vi "水果摊贩子_main.vi"() -> ()   [LabVIEW 2011]
uses:
  <vilib>/Utility/file.llb/Read From Spreadsheet File (string).vi
panel:
  in  "富豪榜":i32[](listbox)
  out "leave":bool
  in  "关闭富豪榜":bool
  in  "查看富豪榜":bool
  in  "退出？":bool
  out "玩家":string caption="请输入你的大名"
  in  "放弃游戏":bool
  out "开心值":dbl(slide) scale=0.0..100.0
  out "当前开心值":i32=1000
  out "提示":string
  in  "银行":bool
  out "存款":i32
  in  "演会中心":bool
  in  "机电学院":bool
  out "天数":i32
  out "余额":i32
  in  "饭堂":bool
  in  "图书馆":bool
  in  "库存":i32[](listbox)
  in  "卖出数量":i32 min=0 step=1
  in  "买入数量":i32 min=0 step=1
  in  "卖出":bool
  in  "买入":bool
  in  "商品价格":i32[](listbox)
  out "物品存在索引":i32[](array[numeric])
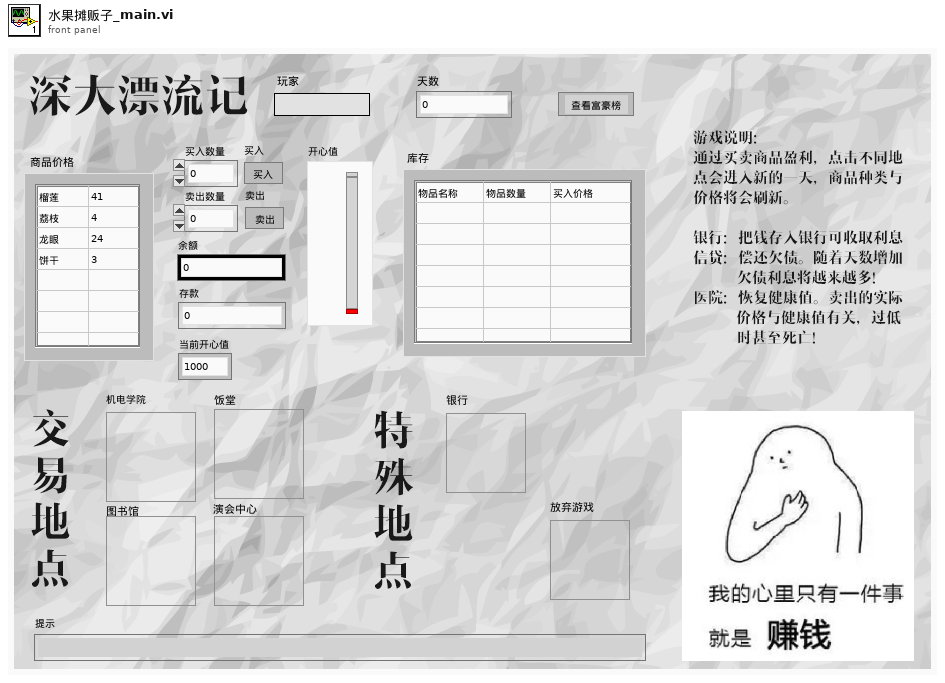
[diagram p1: front panel]
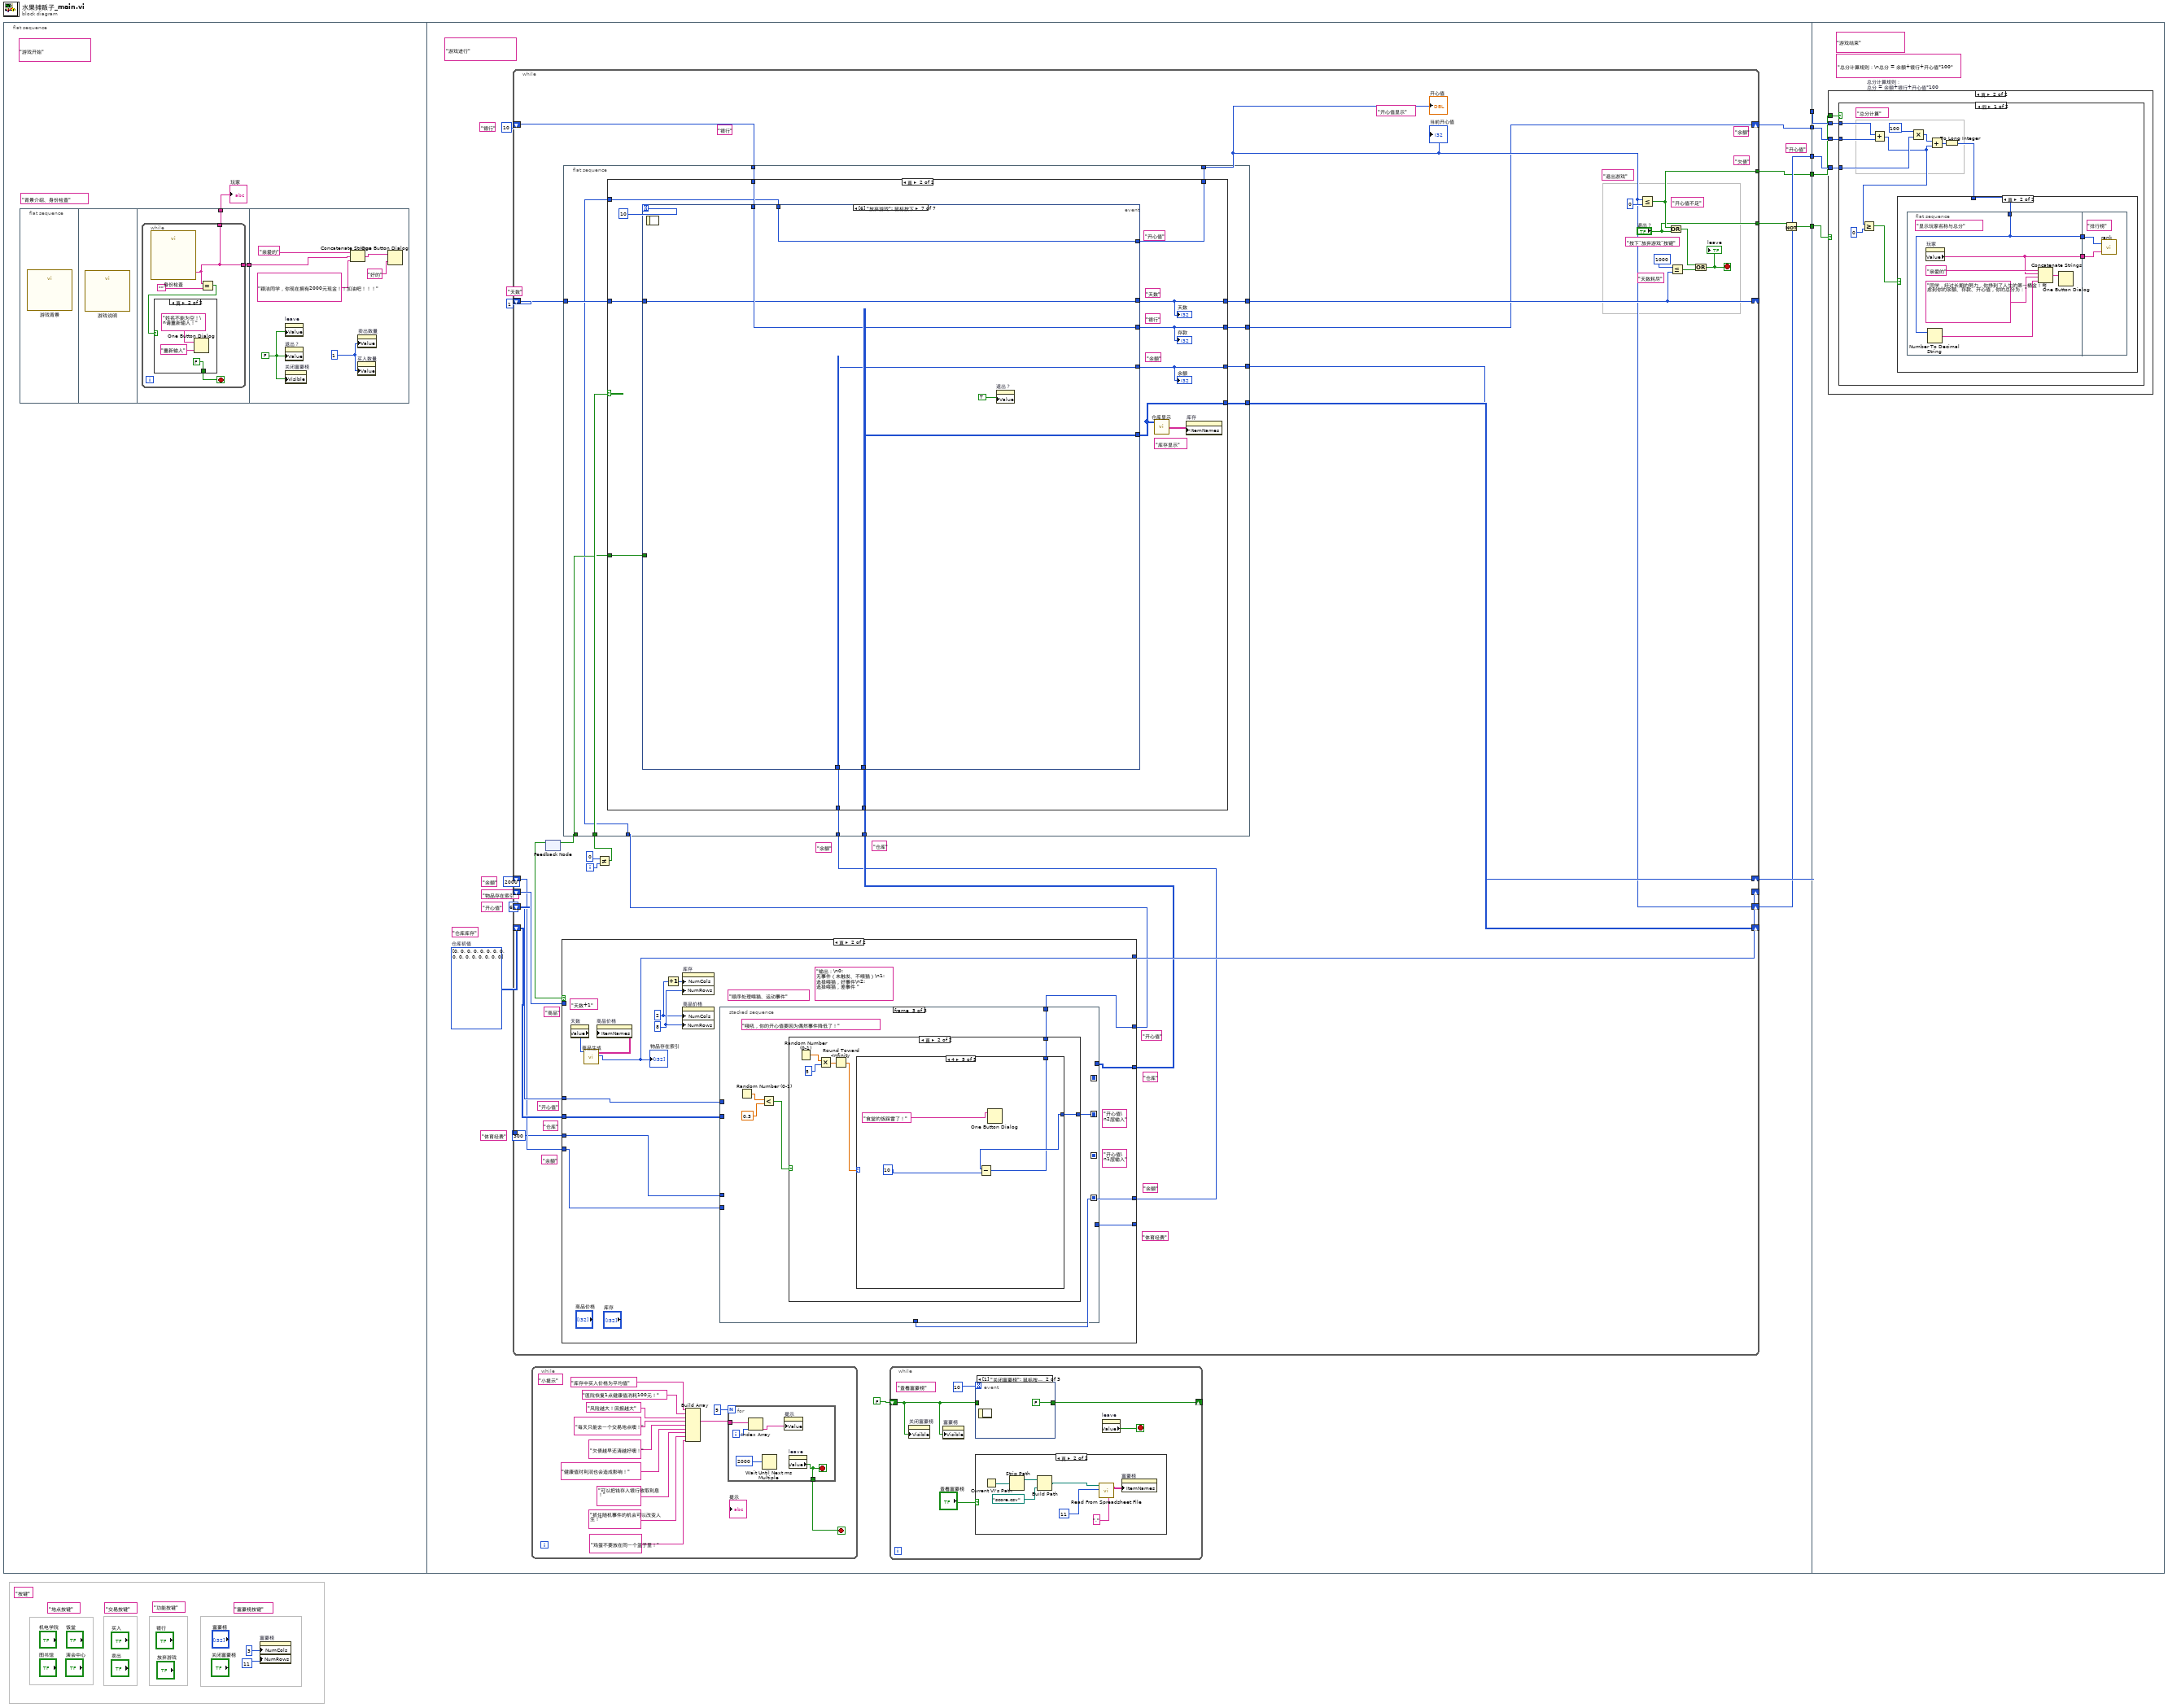
[diagram p0: block diagram]
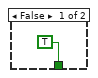
[diagram p2: hidden frame]
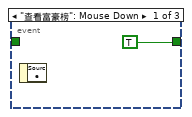
[diagram p3: hidden frame]
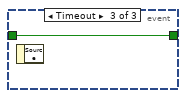
[diagram p4: hidden frame]
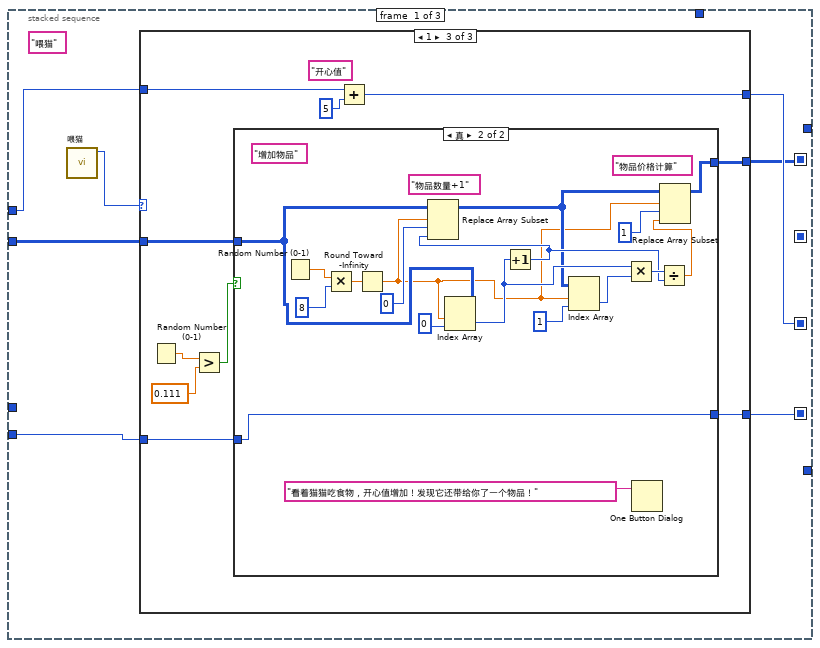
[diagram p7: hidden frame]
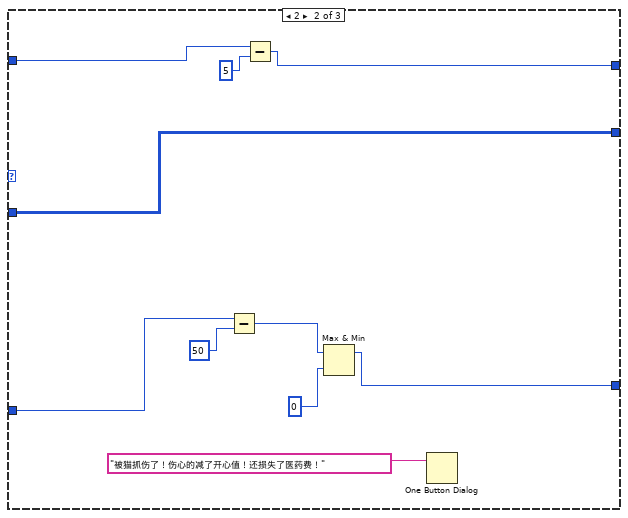
[diagram p9: hidden frame]
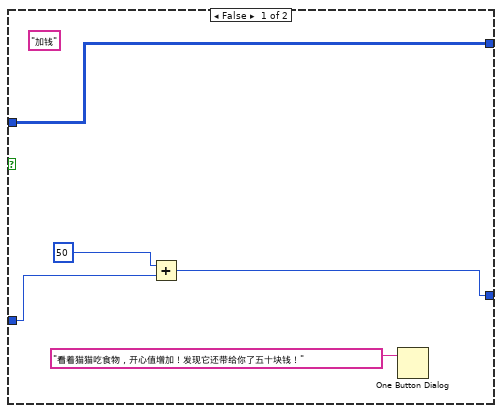
[diagram p10: hidden frame]
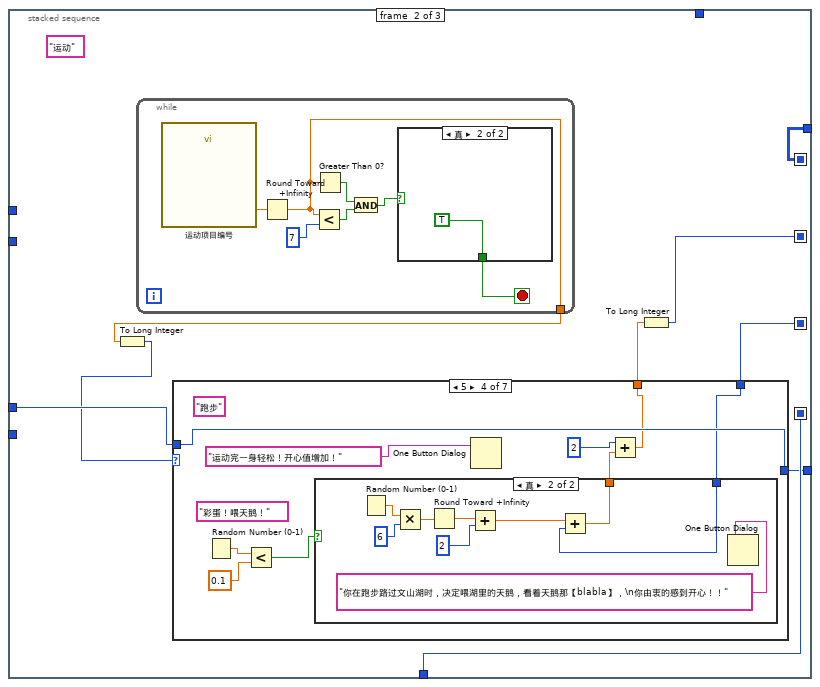
[diagram p11: hidden frame]
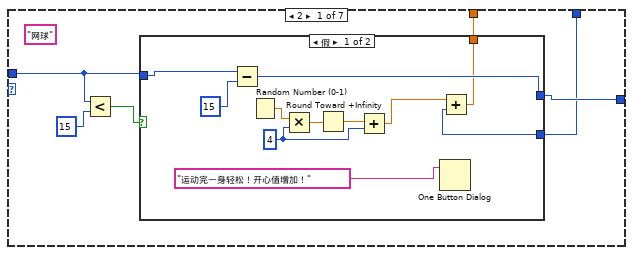
[diagram p12: hidden frame]
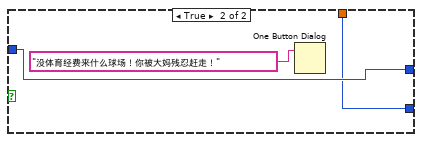
[diagram p13: hidden frame]
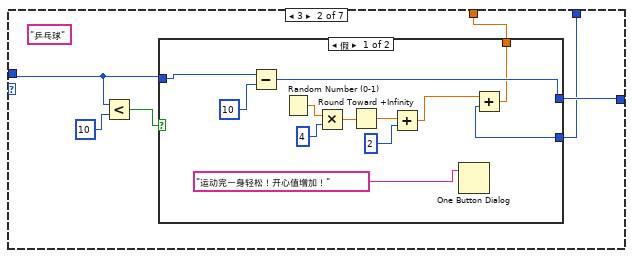
[diagram p14: hidden frame]
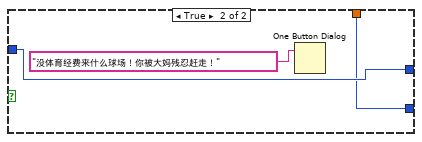
[diagram p15: hidden frame]
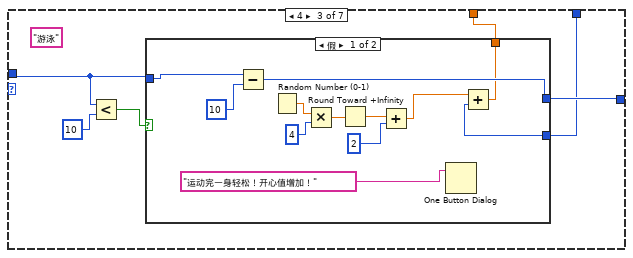
[diagram p16: hidden frame]
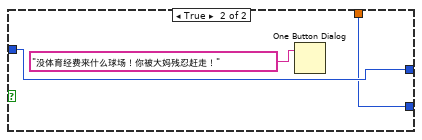
[diagram p17: hidden frame]
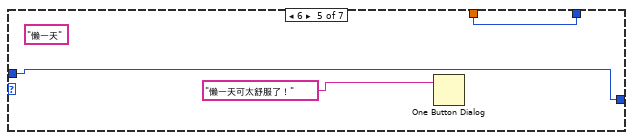
[diagram p19: hidden frame]
diagram:
  (unwired) "富豪榜按键"
  (unwired) "功能按键"
  (unwired) "交易按键"
  (unwired) "地点按键"
  (unwired) "按键"
  n1 = flat-sequence {
    tunnel: [w39] -> w7
    tunnel: [w38] -> w6
    tunnel: [w37] -> w5
    tunnel: [w36] -> w4
    tunnel: [w28] -> w1
    tunnel: w7 -> [w656]
    tunnel: w6 -> [w655]
    tunnel: w5 -> [w654]
    tunnel: w4 -> [w653]
    tunnel: w1 -> [w652]
    frame #0 {
      (unwired) "背景介绍、身份检查"
      (unwired) "游戏开始"
      n2 = flat-sequence {
        tunnel: [w11] -> w9
        tunnel: [w10] -> w8
        tunnel: w9 -> [w25]
        frame #0 {
          n3 = call "游戏背景"() -> ()  [unwired: 18 in, 2 out]
        }
        frame #1 {
          n4 = call "游戏说明"() -> ()  [unwired: 18 in, 2 out]
        }
        frame #2 {
          n5 = while {
            tunnel: [w12] -> w11
            tunnel: [w12] -> w10
            stop <- w13 stop-if-true
            n6 = call "身份检查"() -> ("请输入你的姓名"=w12:string)  [unwired: 17 in, 2 out]
            n7 = Equal?(x=w12, y="") -> (x = y?=w14:bool)
            n8 = case shown="真" w14 {
              tunnel: [TRUE FALSE] -> w13
              frame False {
              }
              frame True {
                n9 = One Button Dialog(message="姓名不能为空！\n请重新输入！", button name ("OK")="重新输入" ("姓名输入提示")) -> ()  [unwired: 1 out]
              }
            }
          }
        }
        frame #3 {
          w20 = 1
          w21 = FALSE
          n10 = property on="leave" class="Bool (严格)"("Value"=w21) -> ()  [unwired: 2 in, 2 out]
          n11 = property on="退出？" class="Bool (严格)"("Value"=w21) -> ()  [unwired: 2 in, 2 out]
          n12 = property on="关闭富豪榜" class="Bool (严格)"("Visible"=w21) -> ()  [unwired: 2 in, 2 out]
          n13 = Concatenate Strings("亲爱的" ("姓名输入提示"), w25, "颖洁同学，你现在拥有2000元现金！！加油吧！！！" ("姓名输入提示")) -> (w23:string)
          n14 = property on="买入数量" class="DigNum (严格)"("Value"=w20) -> ()  [unwired: 2 in, 2 out]
          n15 = property on="卖出数量" class="DigNum (严格)"("Value"=w20) -> ()  [unwired: 2 in, 2 out]
          n16 = One Button Dialog(message=w23, button name ("OK")="好的" ("姓名输入提示")) -> ()  [unwired: 1 out]
        }
      }
      "玩家" <- w8
    }
    frame #1 {
      (unwired) "开心值"
      (unwired) "体育经费"
      (unwired) "物品存在索引"
      (unwired) "游戏进行"
      (unwired) "开心值"
      (unwired) "银行"
      (unwired) "仓库库存"
      (unwired) "天数"
      (unwired) "余额"
      w32 = i32[][] [[0, 0], [0, 0], [0, 0], [0, 0], [0, 0], [0, 0], [0, 0], [0, 0]]  # 仓库初值
      n17 = while {
        shift-right: [w94] -> w39
        shift-left: 2000 -> [w75]
        shift-right: [w95] -> _
        shift-left: w32 -> [w77]
        shift-right: [w98] -> _
        shift-left: _ -> [w97]
        shift-right: [w91] -> _
        shift-left: 1 -> [w88]
        shift-right: [w81] -> w38
        shift-left: 10 -> [w89]
        shift-right: [w82] -> w37
        shift-left: 60 -> [w90]
        tunnel: [w83] -> w36
        tunnel: ["退出？"] -> w29
        tunnel: 300 -> [w72]
        i -> [w93]
        stop <- w86 stop-if-true
        (unwired) "仓库"
        (unwired) "体育经费"
        (unwired) "仓库"
        (unwired) "开心值"
        (unwired) "余额"
        (unwired) "余额"
        (unwired) "天数耗尽"
        (unwired) "按下“放弃游戏”按键"
        (unwired) "开心值不足"
        (unwired) "退出游戏"
        (unwired) "开心值显示"
        (unwired) "开心值"
        (unwired) "余额"
        (unwired) "欠债"
        (unwired) "商品"
        (unwired) "仓库"
        (unwired) "余额"
        (unwired) "银行"
        n18 = feedback-in #1(w80) -> ()
        n19 = feedback #1() -> (w96:bool)  [unwired: 1 in]
        n20 = case shown="真" w96 {
          tunnel: [w104 w114] -> w98
          tunnel: w97 -> [w104 _]
          tunnel: w90 -> [w103 w105]
          tunnel: [w103 w112] -> w73
          tunnel: w77 -> [w102 w111]
          tunnel: [w102 w108] -> w76
          tunnel: w75 -> [w101 w110]
          tunnel: [w101 w109] -> w74
          tunnel: w72 -> [w100 w107]
          tunnel: [w100 w106] -> _
          frame False {
          }
          frame True {
            (unwired) "开心值\n2层输入"
            (unwired) "开心值\n1层输入"
            (unwired) "输出：\n0: 无事件（未触发、不喂猫）\n1: 选择喂猫，好事件\n2: 选择喂猫，差事件 "
            (unwired) "顺序处理喂猫、运动事件"
            (unwired) "天数+1"
            w118 = i8 8
            w116 = i8 2
            n21 = property on="天数" class="DigNum (严格)"() -> ("Value"=w113:i32)  [unwired: 2 in, 2 out]
            n22 = call "商品生成.vi"("天数"=w113) -> ("物品存在索引"=w114:i32[], "市面商品"=w115:string[][])  [unwired: 9 in]
            "物品存在索引" <- w114
            n23 = property on="商品价格" class="MCListbox (严格)"("ItemNames"=w115) -> ()  [unwired: 2 in, 2 out]
            n24 = Increment(x=w116) -> (x+1=w117:i8)
            n25 = property on="库存" class="MCListbox (严格)"("NumCols"=w117, "NumRows"=w118) -> ()  [unwired: 2 in, 2 out]
            n26 = property on="商品价格" class="MCListbox (严格)"("NumCols"=w116, "NumRows"=w118) -> ()  [unwired: 2 in, 2 out]
            n27 = stacked-sequence {
              seq-local: [w124 _ _] -> [_ w177 _]
              seq-local: [w122 _ _] -> [_ w174 _]
              seq-local: [w119 _ _] -> [_ w180 _]
              seq-local: [_ w175 _] -> [_ _ w299]
              tunnel: w105 -> [w125 _ _]
              tunnel: w111 -> [w123 _ _]
              tunnel: w110 -> [w120 _ _]
              tunnel: [_ _ w298] -> w112
              tunnel: [_ w180 _] -> w109
              tunnel: [_ w174 _] -> w108
              tunnel: w107 -> [_ w179 _]
              tunnel: [_ w178 _] -> w106
              frame #0 {
                (unwired) "喂猫"
                n28 = call "喂猫.vi"() -> ("数值"=w121:i8)  [unwired: 11 in]
                n29 = case shown="1" w121 {
                  tunnel: w125 -> [w128 w137 w147]
                  tunnel: [w128 w136 w146] -> w124
                  tunnel: w123 -> [w127 w135 w145]
                  tunnel: [w127 w135 w144] -> w122
                  tunnel: w120 -> [w126 w133 w140]
                  tunnel: [w126 w130 w139] -> w119
                  frame 0, Default {
                  }
                  frame 2 {
                    n30 = Subtract(x=w133, y=50) -> (x-y=w131:i32)
                    n31 = Subtract(x=w137, y=5) -> (x-y=w136:i32)
                    n32 = Max & Min(x=w131, y=0) -> (max(x,y)=w130:i32)  [unwired: 1 out]
                    n33 = One Button Dialog(message="被猫抓伤了！伤心的减了开心值！还损失了医药费！") -> ()  [unwired: 1 in, 1 out]
                  }
                  frame 1 {
                    (unwired) "开心值"
                    n34 = Random Number (0-1)() -> (number: 0 to 1=w143:dbl)
                    n35 = Greater?(x=w143, y=0.111) -> (0:w141:bool)
                    n36 = case shown="真" w141 {
                      tunnel: w145 -> [w153 w166]
                      tunnel: [w153 w156] -> w144
                      tunnel: w140 -> [w152 w155]
                      tunnel: [w150 w155] -> w139
                      frame False {
                        (unwired) "加钱"
                        n37 = Add(x=50, y=w152) -> (x+y=w150:i32)
                        n38 = One Button Dialog(message="看着猫猫吃食物，开心值增加！发现它还带给你了五十块钱！") -> ()  [unwired: 1 in, 1 out]
                      }
                      frame True {
                        (unwired) "物品价格计算"
                        (unwired) "物品数量+1"
                        (unwired) "增加物品"
                        n39 = Random Number (0-1)() -> (number: 0 to 1=w171:dbl)
                        n40 = Multiply(x=w171, y=8) -> (x*y=w169:dbl)
                        n41 = Round Toward -Infinity(1:w169) -> (0:w159:dbl)
                        n42 = Index Array(array=w166, index (row)=w159, index (col)=0) -> (element=w164:i32)
                        n43 = Increment(x=w164) -> (x+1=w161:i32)
                        n44 = Replace Array Subset ("替换数组子集")(array=w166, new element=w161, index (row)=w159, index (col)=0) -> (w160:i32[][])
                        n45 = Index Array(array=w160, index (row)=w159, index (col)=1) -> (element=w167:i32)
                        n46 = Multiply(x=w164, y=w167) -> (x*y=w162:i32)
                        n47 = One Button Dialog(message="看着猫猫吃食物，开心值增加！发现它还带给你了一个物品！") -> ()  [unwired: 1 in, 1 out]
                        n48 = Divide(x=w162, y=w161) -> (x/y=w157:dbl)
                        n49 = Replace Array Subset ("替换数组子集")(array=w160, new element=w157, index (row)=w159, index (col)=1) -> (w156:i32[][])
                      }
                    }
                    n50 = Add(x=w147, y=5) -> (x+y=w146:i32)
                  }
                }
              }
              frame #1 {
                (unwired) "运动"
                n51 = while {
                  tunnel: [w287] -> w173
                  stop <- w288 stop-if-true
                  n52 = call "运动项目编号"() -> ("运动项目"=w293:dbl)  [unwired: 17 in, 2 out]
                  n53 = Round Toward +Infinity(x=w293) -> (ceil(x): smallest int >= x=w287:dbl)
                  n54 = Less?(x=w287, y=7) -> (x < y?=w291:bool)
                  n55 = Greater Than 0?(x=w287) -> (x > 0?=w290:bool)
                  n56 = And(x=w290, y=w291) -> (x .and. y?=w289:bool)
                  n57 = case shown="真" w289 {
                    tunnel: [FALSE TRUE] -> w288
                    frame False {
                      n58 = One Button Dialog(message="输入必须是1-7的整数！", button name ("OK")="重新输入" ("姓名输入提示")) -> ()  [unwired: 1 out]
                    }
                    frame True {
                    }
                  }
                }
                n59 = To Long Integer(number=w173) -> (32bit integer=w172:i32)
                n60 = case shown="5" w172 {
                  tunnel: w179 -> [w183 w203 w224 w251 w263 w265 w269]
                  tunnel: [w184 w204 w225 w251 w263 w265 w270] -> w178
                  tunnel: w177 -> [w182 w202 w223 w246 w262 w266 w268]
                  tunnel: [w181 w201 w222 w243 w262 w266 w267] -> w176
                  frame 2 {
                    (unwired) "网球" ("姓名输入提示")
                    n61 = Less?(x=w183, y=15) -> (x < y?=w185:bool)
                    n62 = case shown="假" w185 {
                      tunnel: w183 -> [w195 w199]
                      tunnel: [w194 w199] -> w184
                      tunnel: w182 -> [w188 w198]
                      tunnel: [w187 w198] -> w181
                      frame False {
                        w190 = 4
                        n63 = Subtract(x=w195, y=15) -> (x-y=w194:i32)
                        n64 = Random Number (0-1)() -> (number: 0 to 1=w193:dbl)
                        n65 = Multiply(x=w193, y=w190) -> (x*y=w192:dbl)
                        n66 = Round Toward +Infinity(x=w192) -> (ceil(x): smallest int >= x=w191:dbl)
                        n67 = Add(x=w191, y=w190) -> (x+y=w189:dbl)
                        n68 = One Button Dialog(message="运动完一身轻松！开心值增加！") -> ()  [unwired: 1 in, 1 out]
                        n69 = Add(x=w189, y=w188) -> (x+y=w187:dbl)
                      }
                      frame True {
                        n70 = One Button Dialog(message="没体育经费来什么球场！你被大妈残忍赶走！") -> ()  [unwired: 1 in, 1 out]
                      }
                    }
                  }
                  frame 3 {
                    (unwired) "乒乓球" ("姓名输入提示")
                    n71 = Less?(x=w203, y=10) -> (x < y?=w206:bool)
                    n72 = case shown="假" w206 {
                      tunnel: w203 -> [w216 w220]
                      tunnel: [w215 w220] -> w204
                      tunnel: w202 -> [w209 w219]
                      tunnel: [w208 w219] -> w201
                      frame False {
                        n73 = Subtract(x=w216, y=10) -> (x-y=w215:i32)
                        n74 = Random Number (0-1)() -> (number: 0 to 1=w214:dbl)
                        n75 = Multiply(x=w214, y=4) -> (x*y=w213:dbl)
                        n76 = Round Toward +Infinity(x=w213) -> (ceil(x): smallest int >= x=w212:dbl)
                        n77 = Add(x=w212, y=2) -> (x+y=w210:dbl)
                        n78 = One Button Dialog(message="运动完一身轻松！开心值增加！") -> ()  [unwired: 1 in, 1 out]
                        n79 = Add(x=w210, y=w209) -> (x+y=w208:dbl)
                      }
                      frame True {
                        n80 = One Button Dialog(message="没体育经费来什么球场！你被大妈残忍赶走！") -> ()  [unwired: 1 in, 1 out]
                      }
                    }
                  }
                  frame 4 {
                    (unwired) "游泳" ("姓名输入提示")
                    n81 = Less?(x=w224, y=10) -> (x < y?=w226:bool)
                    n82 = case shown="假" w226 {
                      tunnel: w224 -> [w237 w241]
                      tunnel: [w236 w241] -> w225
                      tunnel: w223 -> [w230 w240]
                      tunnel: [w229 w240] -> w222
                      frame False {
                        n83 = Subtract(x=w237, y=10) -> (x-y=w236:i32)
                        n84 = Random Number (0-1)() -> (number: 0 to 1=w235:dbl)
                        n85 = Multiply(x=w235, y=4) -> (x*y=w234:dbl)
                        n86 = Round Toward +Infinity(x=w234) -> (ceil(x): smallest int >= x=w233:dbl)
                        n87 = Add(x=w233, y=2) -> (x+y=w231:dbl)
                        n88 = One Button Dialog(message="运动完一身轻松！开心值增加！") -> ()  [unwired: 1 in, 1 out]
                        n89 = Add(x=w231, y=w230) -> (x+y=w229:dbl)
                      }
                      frame True {
                        n90 = One Button Dialog(message="没体育经费来什么球场！你被大妈残忍赶走！") -> ()  [unwired: 1 in, 1 out]
                      }
                    }
                  }
                  frame 5 {
                    (unwired) "彩蛋！喂天鹅！"
                    (unwired) "跑步" ("姓名输入提示")
                    n91 = Random Number (0-1)() -> (number: 0 to 1=w249:dbl)
                    n92 = Less?(x=w249, y=0.1) -> (x < y?=w247:bool)
                    n93 = case shown="真" w247 {
                      tunnel: w246 -> [w252 w254]
                      tunnel: [w252 w253] -> w245
                      frame False {
                      }
                      frame True {
                        n94 = Random Number (0-1)() -> (number: 0 to 1=w260:dbl)
                        n95 = Multiply(x=w260, y=6) -> (x*y=w259:dbl)
                        n96 = Round Toward +Infinity(x=w259) -> (ceil(x): smallest int >= x=w258:dbl)
                        n97 = Add(x=w258, y=2) -> (x+y=w255:dbl)
                        n98 = Add(x=w255, y=w254) -> (x+y=w253:dbl)
                        n99 = One Button Dialog(message="你在跑步路过文山湖时，决定喂湖里的天鹅，看着天鹅那【blabla】，\n你由衷的感到开心！！") -> ()  [unwired: 1 in, 1 out]
                      }
                    }
                    n100 = One Button Dialog(message="运动完一身轻松！开心值增加！") -> ()  [unwired: 1 in, 1 out]
                    n101 = Add(x=2, y=w245) -> (x+y=w243:dbl)
                  }
                  frame 6 {
                    (unwired) "懒一天" ("姓名输入提示")
                    n102 = One Button Dialog(message="懒一天可太舒服了！") -> ()  [unwired: 1 in, 1 out]
                  }
                  frame 7, Default {
                  }
                  frame 1 {
                    (unwired) "羽毛球" ("姓名输入提示")
                    n103 = Less?(x=w269, y=15) -> (x < y?=w271:bool)
                    n104 = case shown="假" w271 {
                      tunnel: w269 -> [w281 w285]
                      tunnel: [w280 w285] -> w270
                      tunnel: w268 -> [w275 w284]
                      tunnel: [w273 w284] -> w267
                      frame False {
                        w276 = 4
                        n105 = Subtract(x=w281, y=15) -> (x-y=w280:i32)
                        n106 = Random Number (0-1)() -> (number: 0 to 1=w279:dbl)
                        n107 = Multiply(x=w279, y=w276) -> (x*y=w278:dbl)
                        n108 = Round Toward +Infinity(x=w278) -> (ceil(x): smallest int >= x=w277:dbl)
                        n109 = Add(x=w277, y=w276) -> (x+y=w274:dbl)
                        n110 = One Button Dialog(message="运动完一身轻松！开心值增加！") -> ()  [unwired: 1 in, 1 out]
                        n111 = Add(x=w274, y=w275) -> (x+y=w273:dbl)
                      }
                      frame True {
                        n112 = One Button Dialog(message="没体育经费来什么球场！你被大妈残忍赶走！") -> ()  [unwired: 1 in, 1 out]
                      }
                    }
                  }
                }
                n113 = To Long Integer(number=w176) -> (32bit integer=w175:i32)
              }
              frame #2 {
                (unwired) "哦吼，你的开心值要因为偶然事件降低了！"
                n114 = Random Number (0-1)() -> (number: 0 to 1=w302:dbl)
                n115 = Less?(x=w302, y=0.3) -> (x < y?=w300:bool)
                n116 = case shown="真" w300 {
                  tunnel: w299 -> [w303 w305]
                  tunnel: [w303 w304] -> w298
                  frame False {
                  }
                  frame True {
                    n117 = Random Number (0-1)() -> (number: 0 to 1=w308:dbl)
                    n118 = Multiply(x=w308, y=5) -> (x*y=w307:dbl)
                    n119 = Round Toward -Infinity(1:w307) -> (0:w306:dbl)
                    n120 = case shown="4" w306 {
                      tunnel: w305 -> [w311 w315 w319 w323 w327]
                      tunnel: [w310 w314 w318 w322 w326] -> w304
                      frame 0, Default {
                        n121 = Subtract(x=w311, y=30) -> (x-y=w310:i32)
                        n122 = One Button Dialog(message="导师催PPT啦！难过的哭出来！") -> ()  [unwired: 1 in, 1 out]
                      }
                      frame 1 {
                        n123 = Subtract(x=w315, y=20) -> (x-y=w314:i32)
                        n124 = One Button Dialog(message="今天生病了！开心值下降！") -> ()  [unwired: 1 in, 1 out]
                      }
                      frame 2 {
                        n125 = Subtract(x=w319, y=20) -> (x-y=w318:i32)
                        n126 = One Button Dialog(message="热水器又坏了！！！！") -> ()  [unwired: 1 in, 1 out]
                      }
                      frame 3 {
                        n127 = Subtract(x=w323, y=10) -> (x-y=w322:i32)
                        n128 = One Button Dialog(message="今天要手洗外套啦！") -> ()  [unwired: 1 in, 1 out]
                      }
                      frame 4 {
                        n129 = Subtract(x=w327, y=10) -> (x-y=w326:i32)
                        n130 = One Button Dialog(message="食堂的饭踩雷了！") -> ()  [unwired: 1 in, 1 out]
                      }
                    }
                  }
                }
              }
            }
          }
        }
        n131 = flat-sequence "平铺式顺序结构" {
          tunnel: w74 -> [w341]
          tunnel: [w337] -> w94
          tunnel: w79 -> [w340]
          tunnel: w76 -> [w339]
          tunnel: [w336] -> w95
          tunnel: [w338] -> w80
          tunnel: [w335] -> w91
          tunnel: w89 -> [w333]
          tunnel: [w332] -> w81
          tunnel: [w331] -> w82
          tunnel: w73 -> [w330]
          tunnel: w88 -> [w334]
          frame #0 {
            n132 = case shown="真" w340 {
              tunnel: w341 -> [w347 w354]
              tunnel: [w347 w350] -> w337
              tunnel: w339 -> [w346 w348]
              tunnel: [w346 w358] -> w336
              tunnel: [TRUE w360] -> w338
              tunnel: [w344 w349] -> w335
              tunnel: w334 -> [w344 w356]
              tunnel: w333 -> [w343 w355]
              tunnel: [w343 w351] -> w332
              tunnel: [w342 w353] -> w331
              tunnel: w330 -> [w342 w352]
              frame False {
              }
              frame True {
                (unwired) "库存显示"
                (unwired) "余额"
                (unwired) "天数"
                (unwired) "开心值"
                (unwired) "银行"
                n133 = event shown="[6] \"放弃游戏\": 鼠标按下" {
                  selector: _ -> [_ _ _ _ _ _ _]
                  dyn-events: _ -> [_ _ _ _ _ _ _]
                  timeout: 10 -> [_ _ _ _ _ _ _]
                  tunnel: [w364 w372 w452 w578 w586 w589 w648] -> w350
                  tunnel: w354 -> [w364 w369 w453 w578 w586 w593 w648]
                  tunnel: [w365 w373 w450 w579 w585 w590 w651] -> w358
                  tunnel: [FALSE FALSE _ TRUE FALSE _ _] -> w360
                  tunnel: w348 -> [w365 w374 w451 w579 w585 w590 w651]
                  tunnel: [w363 w370 w448 w574 w583 w588 w647] -> w349
                  tunnel: w356 -> [w363 w370 w448 w576 w583 w588 w647]
                  tunnel: w355 -> [w362 w368 w449 w570 w582 w592 w649]
                  tunnel: [w362 w368 w449 w571 w582 w591 w649] -> w351
                  tunnel: w352 -> [w361 w367 w447 w575 w581 w587 w650]
                  tunnel: [w361 w367 w447 w575 w581 w587 w650] -> w353
                  event Timeout {
                    n134 = event-data() -> ()  [unwired: 1 in, 3 out]
                  }
                  event "买入": Mouse Down {
                    n135 = event-data() -> ()  [unwired: 1 in, 1 out]
                    n136 = stacked-sequence {
                      seq-local: ["买入数量" _] -> [_ w387]
                      seq-local: [w377 _] -> [_ w388]
                      seq-local: [w376 _] -> [_ w384]
                      seq-local: [w375 _] -> [_ w385]
                      tunnel: w369 -> [_ w392]
                      tunnel: w374 -> [_ w391]
                      tunnel: [_ w390] -> w373
                      tunnel: [_ w389] -> w372
                      frame #0 {
                        (unwired) "使用顺序结构，确保物品价格与买入数量为最新参数"
                        (unwired) "买入数量"
                        (unwired) "买入物品价格"
                        n137 = property on="商品价格" class="MCListbox (严格)"() -> ("ItemNames"=w380:string[][], "Value"=w379:i32[])  [unwired: 2 in, 2 out]
                        n138 = Index Array(array=w379, index=0) -> (element=w376:i32)
                        n139 = Index Array(array=w380, index (row)=w376) -> (element=w381:string[])  [unwired: 1 in]
                        n140 = Index Array(array=w381, index=1) -> (element=w375:string)
                        n141 = Decimal String To Number(string=w375) -> (number=w377:i32)  [unwired: 2 in, 1 out]
                      }
                      frame #1 {
                        (unwired) "判断买入数量是否小于零"
                        n142 = Greater Than 0?(x=w387) -> (x > 0?=w386:bool)
                        n143 = case shown="真" w386 {
                          tunnel: w392 -> [w394 w397]
                          tunnel: w385 -> [_ w405]
                          tunnel: w384 -> [_ w404]
                          tunnel: w391 -> [w393 w403]
                          tunnel: [w393 w402] -> w390
                          tunnel: [w394 w401] -> w389
                          tunnel: w388 -> [_ w400]
                          tunnel: w387 -> [_ w396]
                          frame False {
                            n144 = One Button Dialog(message="买入数量不能小于零！！") -> ()  [unwired: 1 in, 1 out]
                          }
                          frame True {
                            (unwired) "计算余额"
                            n145 = Multiply(x=w400, y=w396) -> (x*y=w406:i32)
                            n146 = Subtract(x=w397, y=w406) -> (x-y=w399:i32)
                            n147 = Less Than 0?(x=w399) -> (x < 0?=w398:bool)
                            n148 = case shown="假" w398 {
                              tunnel: [w430 w446] -> w401
                              tunnel: w399 -> [w430 _]
                              tunnel: w397 -> [_ w446]
                              tunnel: w405 -> [w424 _]
                              tunnel: w404 -> [w411 _]
                              tunnel: w403 -> [w407 w445]
                              tunnel: [w417 w445] -> w402
                              tunnel: w396 -> [w413 _]
                              tunnel: w396 -> [w410 _]
                              frame False {
                                (unwired) "更新物品数量与均价"
                                (unwired) "计算买入均价"
                                (unwired) "获取索引位置"
                                n149 = property on="物品存在索引" class="Arr (严格)"() -> ("Value"=w408:i32[])  [unwired: 2 in, 2 out]
                                n150 = for {
                                N: 8 -> [_]
                                tunnel: w408 -> [w440]
                                shift-right: [w436] -> _
                                shift-left: 0 -> [w437]
                                tunnel: w411 -> [w434]
                                tunnel: [w433] -> w409
                                i -> [w433]
                                stop <- w431 stop-if-true
                                n151 = Index Array(array=w440, index=w433) -> (element=w439:i32)
                                n152 = Equal?(x=w439, y=1) -> (x = y?=w432:bool)
                                n153 = case shown="真" w432 {
                                tunnel: w437 -> [w441 w443]
                                tunnel: [w441 w442] -> w436
                                frame False {
                                }
                                frame True {
                                n154 = Increment(x=w443) -> (x+1=w442:i32)
                                }
                                }
                                n155 = Decrement(x=w436) -> (x-1=w435:i32)
                                n156 = Equal?(x=w434, y=w435) -> (x = y?=w431:bool)
                                }
                                n157 = Decimal String To Number(string=w424) -> (number=w423:i32)  [unwired: 2 in, 1 out]
                                n158 = Index Array(array=w407, index (row) #1=w409, index (col) #1=0, index (row) #2=w409, index (col) #2=1) -> (element #1=w420:i32, element #2=w425:i32)
                                n159 = Multiply(x=w420, y=w425) -> (x*y=w422:i32)
                                n160 = Add(x=w420, y=w410) -> (x+y=w418:i32)
                                n161 = Add(x=w413, y=w420) -> (x+y=w427:i32)
                                n162 = Multiply(x=w423, y=w410) -> (x*y=w421:i32)
                                n163 = Add(x=w422, y=w421) -> (x+y=w419:i32)
                                n164 = Divide(x=w419, y=w418) -> (x/y=w414:dbl)
                                n165 = Replace Array Subset(array=w407, new element #1=w427, index (row) #1=w409, index (col) #1=0, new element #2=w414, index (row) #2=w409, index (col) #2=1) -> (w417:i32[][])
                              }
                              frame True {
                                n166 = One Button Dialog(message="余额不足！请重新输入") -> ()  [unwired: 1 in, 1 out]
                              }
                            }
                          }
                        }
                      }
                    }
                  }
                  event "卖出": Mouse Down {
                    n167 = event-data() -> ()  [unwired: 1 in, 1 out]
                    n168 = stacked-sequence {
                      seq-local: ["卖出数量" _] -> [_ w463]
                      seq-local: [w459 _] -> [_ w471]
                      seq-local: [w454 _] -> [_ w467]
                      tunnel: w451 -> [_ w470]
                      tunnel: w453 -> [_ w469]
                      tunnel: [_ w468] -> w452
                      tunnel: [_ w466] -> w450
                      tunnel: w447 -> [_ w465]
                      frame #0 {
                        n169 = property on="库存" class="MCListbox (严格)"() -> ("ItemNames"=w457:string[][], "Value"=w456:i32[])  [unwired: 2 in, 2 out]
                        n170 = Index Array(array=w456, index=0) -> (element=w454:i32)
                        n171 = Index Array(array=w457, index (row)=w454) -> (element=w458:string[])  [unwired: 1 in]
                        n172 = Index Array(array=w458, index=1) -> (element=w460:string)
                        n173 = Decimal String To Number(string=w460) -> (number=w459:i32)  [unwired: 2 in, 1 out]
                      }
                      frame #1 {
                        (unwired) "库存\n索引"
                        (unwired) "库存\n数量"
                        (unwired) "卖出\n数量"
                        (unwired) "判断卖出数量是否大于零"
                        n174 = Greater Or Equal To 0?(x=w463) -> (x >= 0?=w464:bool)
                        n175 = case shown="真" w464 {
                          tunnel: w471 -> [_ w484]
                          tunnel: w470 -> [w472 w482]
                          tunnel: w469 -> [w473 w481]
                          tunnel: [w473 w480] -> w468
                          tunnel: w467 -> [_ w479]
                          tunnel: w463 -> [_ w477]
                          tunnel: [w472 w476] -> w466
                          tunnel: w465 -> [_ w475]
                          frame False {
                            n176 = One Button Dialog(message="卖出数量不能为负数！！！") -> ()  [unwired: 1 in, 1 out]
                          }
                          frame True {
                            (unwired) "判断是否选中商品"
                            n177 = Less?(x=w484, y=w477) -> (x < y?=w483:bool)
                            n178 = Not Equal To 0?(x=w479) -> (x != 0?=w478:bool)
                            n179 = case shown="真" w478 {
                              tunnel: w483 -> [_ w491]
                              tunnel: w482 -> [w485 w495]
                              tunnel: w479 -> [_ w494]
                              tunnel: w477 -> [_ w493]
                              tunnel: w481 -> [w486 w488]
                              tunnel: [w486 w492] -> w480
                              tunnel: [w485 w490] -> w476
                              tunnel: w475 -> [_ w489]
                              frame False {
                                n180 = One Button Dialog(message="没有选中商品！请重新选择~") -> ()  [unwired: 1 in, 1 out]
                              }
                              frame True {
                                (unwired) "判断卖出数量是否超过库存量"
                                n181 = case shown="假" w491 {
                                tunnel: w495 -> [w501 w568]
                                tunnel: w494 -> [w506 _]
                                tunnel: w493 -> [w496 _]
                                tunnel: [w502 w567] -> w492
                                tunnel: [w499 w568] -> w490
                                tunnel: w489 -> [w498 _]
                                tunnel: w488 -> [w497 w567]
                                frame False {
                                (unwired) "判断市面中是否存在卖出商品"
                                (unwired) "索引所选择商品"
                                n182 = for {
                                N: 8 -> [_]
                                tunnel: w501 -> [w559]
                                shift-right: [w561] -> _
                                shift-left: 0 -> [w557]
                                tunnel: w506 -> [w558]
                                tunnel: [w556] -> w500
                                i -> [w556]
                                stop <- w560 stop-if-true
                                n183 = Index Array(array=w559, index (row)=w556, index (col)=0) -> (element=w563:i32)
                                n184 = Not Equal To 0?(x=w563) -> (x != 0?=w562:bool)
                                n185 = case shown="真" w562 {
                                tunnel: [w564 w566] -> w561
                                tunnel: w557 -> [w564 w565]
                                frame False {
                                }
                                frame True {
                                n186 = Increment(x=w565) -> (x+1=w566:i32)
                                }
                                }
                                n187 = Equal?(x=w561, y=w558) -> (x = y?=w560:bool)
                                }
                                n188 = property on="物品存在索引" class="Arr (严格)"() -> ("Value"=w503:i32[])  [unwired: 2 in, 2 out]
                                n189 = Index Array(array=w503, index=w500) -> (element=w505:i32)
                                n190 = Not Equal To 0?(x=w505) -> (x != 0?=w504:bool)
                                n191 = case shown="真" w504 {
                                tunnel: w500 -> [_ w542]
                                tunnel: w503 -> [_ w543]
                                tunnel: w496 -> [_ w523]
                                tunnel: w497 -> [w510 w537]
                                tunnel: [w510 w536] -> w502
                                tunnel: w501 -> [_ w534]
                                tunnel: w500 -> [_ w533]
                                tunnel: w496 -> [_ w531]
                                tunnel: w501 -> [w509 w528]
                                tunnel: w500 -> [_ w527]
                                tunnel: [w509 w526] -> w499
                                tunnel: w498 -> [_ w522]
                                frame False {
                                n192 = One Button Dialog(message="黑市并没有该商品的交易！先屯着吧~") -> ()  [unwired: 1 in, 1 out]
                                }
                                frame True {
                                (unwired) "判断库存是否卖完"
                                (unwired) "去除库存"
                                (unwired) "余额计算"
                                n193 = property on="商品价格" class="MCListbox (严格)"() -> ("ItemNames"=w540:string[][])  [unwired: 2 in, 2 out]
                                n194 = Array Subset(array=w543, length=w542) -> (w541:i32[])  [unwired: 1 in]
                                n195 = Index Array(array=w534, index (row)=w533, index (col)=0) -> (element=w530:i32)
                                n196 = Add Array Elements(numeric array=w541) -> (sum=w539:i32)
                                n197 = Subtract(x=w530, y=w531) -> (x-y=w525:i32)
                                n198 = Equal To 0?(x=w525) -> (x = 0?=w529:bool)
                                n199 = Index Array(array=w540, index (row)=w539, index (col)=1) -> (element=w524:string)
                                n200 = case shown="假" w529 {
                                tunnel: w528 -> [w549 w554]
                                tunnel: w527 -> [w548 w553]
                                tunnel: [w545 w550] -> w526
                                tunnel: w525 -> [w546 _]
                                frame False {
                                n201 = Replace Array Subset(array=w549, new element=w546, index (row)=w548, index (col)=0) -> (w545:i32[][])
                                }
                                frame True {
                                w551 = 0
                                n202 = Increment(x=w551) -> (x+1=w552:i32)
                                n203 = Replace Array Subset(array=w554, new element #1=w551, index (row) #1=w553, index (col) #1=w551, new element #2=w551, index (row) #2=w553, index (col) #2=w552) -> (w550:i32[][])
                                }
                                }
                                n204 = Decimal String To Number(string=w524) -> (number=w535:i32)  [unwired: 2 in, 1 out]
                                n205 = Multiply(x=w535, y=w523) -> (x*y=w515:i32)
                                n206 = Quotient & Remainder(x=w522, y=100) -> (floor(x/y)=w512:i32)  [unwired: 1 out]
                                n207 = Decrement(x=w512) -> (x-1=w514:i32)
                                n208 = Greater Than 0?(x=w514) -> (x > 0?=w513:bool)
                                n209 = Multiply(x=w512, y=0.1) -> (x*y=w518:dbl)
                                n210 = case shown="真" w513 {
                                frame False {
                                }
                                frame True {
                                n211 = One Button Dialog(message="满满的开心值让你在与买家的谈判中游刃有余，卖出价格超过市面价格！") -> ()  [unwired: 1 in, 1 out]
                                }
                                }
                                n212 = Increment(x=w518) -> (x+1=w516:dbl)
                                n213 = Multiply(x=w516, y=w515) -> (x*y=w517:dbl)
                                n214 = To Long Integer(number=w517) -> (32bit integer=w519:i32)
                                n215 = Add(x=w519, y=w537) -> (x+y=w536:i32)
                                }
                                }
                                }
                                frame True {
                                n216 = One Button Dialog(message="库存太少啦！请重新选择~") -> ()  [unwired: 1 in, 1 out]
                                }
                                }
                              }
                            }
                          }
                        }
                      }
                    }
                  }
                  event "图书馆", "机电学院", "演会中心", "饭堂": Mouse Up {
                    n217 = event-data() -> ()  [unwired: 1 in, 8 out]
                    n218 = Add(x=1, y=w576) -> (x+y=w574:i32)
                    n219 = Multiply(x=w570, y=1.05) -> (x*y=w572:dbl)
                    n220 = To Long Integer(number=w572) -> (32bit integer=w571:i32)
                  }
                  event "库存", "商品价格": Mouse Down {
                    n221 = event-data() -> ()  [unwired: 1 in, 8 out]
                  }
                  event "银行": Mouse Down {
                    n222 = event-data() -> ()  [unwired: 1 in, 1 out]
                    n223 = Two Button Dialog(message="欢迎来到 IronBank ，你打算干什么？", 1:"取款", 2:"存款") -> (T button?=w594:bool)
                    n224 = case shown="真" w594 {
                      tunnel: w593 -> [w604 w628]
                      tunnel: w592 -> [w603 w627]
                      tunnel: [w602 w626] -> w589
                      tunnel: [w601 w625] -> w591
                      frame False {
                        (unwired) "取款"
                        n225 = call "输入取款数额"() -> ("取款数额"=w599:dbl)  [unwired: 17 in, 2 out]
                        n226 = To Long Integer(number=w599) -> (32bit integer=w598:i32)
                        n227 = Greater Or Equal To 0?(x=w598) -> (x >= 0?=w600:bool)
                        n228 = case shown="真" w600 {
                          tunnel: w604 -> [w607 w612]
                          tunnel: w603 -> [w606 w609]
                          tunnel: [w606 w611] -> w602
                          tunnel: [w607 w610] -> w601
                          tunnel: w598 -> [_ w608]
                          frame False {
                            n229 = One Button Dialog(message="取款数额必须大于等于0！") -> ()  [unwired: 1 in, 1 out]
                          }
                          frame True {
                            n230 = Less?(x=w609, y=w608) -> (x < y?=w613:bool)
                            n231 = case shown="假" w613 {
                              tunnel: [w618 w619] -> w611
                              tunnel: [w617 w620] -> w610
                              tunnel: w608 -> [w616 _]
                              tunnel: w612 -> [w615 w619]
                              tunnel: w609 -> [w614 w620]
                              frame False {
                                n232 = Subtract(x=w614, y=w616) -> (x-y=w617:i32)
                                n233 = Add(x=w615, y=w616) -> (x+y=w618:i32)
                              }
                              frame True {
                                n234 = One Button Dialog(message="余额不足！请重新输入") -> ()  [unwired: 1 in, 1 out]
                              }
                            }
                          }
                        }
                      }
                      frame True {
                        (unwired) "存款"
                        n235 = call "输入存款数额"() -> ("存款数额"=w623:dbl)  [unwired: 17 in, 2 out]
                        n236 = To Long Integer(number=w623) -> (32bit integer=w622:i32)
                        n237 = Greater Or Equal To 0?(x=w622) -> (x >= 0?=w624:bool)
                        n238 = case shown="真" w624 {
                          tunnel: w628 -> [w629 w636]
                          tunnel: w627 -> [w630 w635]
                          tunnel: [w629 w634] -> w626
                          tunnel: [w630 w633] -> w625
                          tunnel: w622 -> [_ w632]
                          frame False {
                            n239 = One Button Dialog(message="存款数额必须大于等于0！") -> ()  [unwired: 1 in, 1 out]
                          }
                          frame True {
                            n240 = Less?(x=w636, y=w632) -> (x < y?=w637:bool)
                            n241 = case shown="假" w637 {
                              tunnel: w632 -> [w642 _]
                              tunnel: [w641 w644] -> w634
                              tunnel: [w640 w643] -> w633
                              tunnel: w636 -> [w639 w644]
                              tunnel: w635 -> [w638 w643]
                              frame False {
                                n242 = Add(x=w638, y=w642) -> (x+y=w640:i32)
                                n243 = Subtract(x=w639, y=w642) -> (x-y=w641:i32)
                              }
                              frame True {
                                n244 = One Button Dialog(message="余额不足！请重新输入") -> ()  [unwired: 1 in, 1 out]
                              }
                            }
                          }
                        }
                      }
                    }
                  }
                  event "放弃游戏": Mouse Down {
                    n245 = event-data() -> ()  [unwired: 1 in, 1 out]
                    n246 = property on="退出？" class="Bool (严格)"("Value"=TRUE) -> ()  [unwired: 2 in, 2 out]
                  }
                }
                "余额" <- w350
                "天数" <- w349
                "存款" <- w351
                n247 = call "仓库显示.vi"("仓库"=w358) -> ("显示栏"=w357:string[][])  [unwired: 10 in]
                n248 = property on="库存" class="MCListbox (严格)"("ItemNames"=w357) -> ()  [unwired: 2 in, 2 out]
              }
            }
          }
        }
        n249 = Not Equal?(x=0, y=w93) -> (x != y?=w79:bool)
        n250 = Less Or Equal?(x=w82, y=0) -> (x <= y?=w83:bool)
        n251 = Or(x=w83, y="退出？") -> (x .or. y?=w84:bool)
        n252 = Less Or Equal?(x=1000, y=w91) -> (x <= y?=w87:bool)
        n253 = Or(x=w84, y=w87) -> (x .or. y?=w86:bool)
        "leave" <- w86
        "当前开心值" <- w82
        "开心值" <- w82
      }
      n254 = while {
        stop <- w43 stop-if-true
        (unwired) "小提示"
        n255 = Build Array("库存中买入价格为平均值", "医院恢复1点健康值消耗100元！", "风险越大！回报越大", "每天只能去一个交易地点噢！", "欠债越早还清越好噢！", "健康值对利润也会造成影响！", "可以把钱存入银行收取利息！", "抓住随机事件的机会可以改变人生！", "鸡蛋不要放在同一个篮子里！") -> (w51:string[])
        n256 = for {
          N: 9 -> [_]
          tunnel: w51 -> [w56]
          tunnel: [w52] -> w43
          i -> [w55]
          stop <- w52 stop-if-true
          n257 = Index Array(array=w56, index=w55) -> (element=w53:string)
          n258 = Wait Until Next ms Multiple(millisecond multiple=2000) -> ()  [unwired: 1 out]
          n259 = property on="提示" class="Str"("Value"=w53) -> ()  [unwired: 2 in, 2 out]
          n260 = property on="leave" class="Bool (严格)"() -> ("Value"=w52:bool)  [unwired: 2 in, 2 out]
        }
      }
      n261 = while {
        shift-right: [w58] -> _
        shift-left: FALSE -> [w57]
        stop <- w59 stop-if-true
        (unwired) "查看富豪榜"
        n262 = property on="关闭富豪榜" class="Bool (严格)"("Visible"=w57) -> ()  [unwired: 2 in, 2 out]
        n263 = property on="富豪榜" class="MCListbox (严格)"("Visible"=w57) -> ()  [unwired: 2 in, 2 out]
        n264 = event shown="[1] \"关闭富豪榜\": 鼠标按下" {
          selector: _ -> [_ _ _]
          dyn-events: _ -> [_ _ _]
          timeout: 10 -> [_ _ _]
          tunnel: w57 -> [_ _ w64]
          tunnel: [TRUE FALSE w64] -> w58
          event "查看富豪榜": Mouse Down {
            n265 = event-data() -> ()  [unwired: 1 in, 1 out]
          }
          event "关闭富豪榜": Mouse Down {
            n266 = event-data() -> ()  [unwired: 1 in, 1 out]
          }
          event Timeout {
            n267 = event-data() -> ()  [unwired: 1 in, 1 out]
          }
        }
        n268 = case shown="真" "查看富豪榜" {
          frame False {
          }
          frame True {
            n269 = Current VI's Path() -> (path=w69:path)
            n270 = Strip Path(path=w69) -> (stripped path=w68:path)  [unwired: 1 out]
            n271 = Build Path(base path=w68, name or relative path=path "score.csv") -> (appended path=w66:path)
            n272 = call-poly <vilib>:"Read From Spreadsheet File.vi"("delimiter (\\t)"=",", "number of rows (all:-1)"=11, "file path (dialog if empty)"=w66) -> ("all rows"=w65:string[][])  [unwired: 4 in, 4 out]
            n273 = property on="富豪榜" class="MCListbox (严格)"("ItemNames"=w65) -> ()  [unwired: 2 in, 2 out]
          }
        }
        n274 = property on="leave" class="Bool (严格)"() -> ("Value"=w59:bool)  [unwired: 2 in, 2 out]
      }
      n275 = Not(x=w29) -> (.not. x?=w28:bool)
    }
    frame #2 {
      (unwired) "总分计算规则：\n总分 = 余额+银行+开心值*100"  # 总分计算规则： 总分 = 余额+银行+开心值*100
      (unwired) "游戏结束"
      n276 = case shown="真" w652 {
        tunnel: w656 -> [_ w664]
        tunnel: w655 -> [_ w663]
        tunnel: w654 -> [_ w662]
        tunnel: w653 -> [_ w661]
        frame False {
          n277 = property on="玩家" class="Str"() -> ("Value"=w657:string)  [unwired: 2 in, 2 out]
          n278 = Concatenate Strings("亲爱的", w657, "同学，你点击了放弃游戏！重新开始请点击”运行“按钮！") -> (w658:string)
          n279 = One Button Dialog(message=w658) -> ()  [unwired: 1 in, 1 out]
        }
        frame True {
          n280 = case shown="假" w661 {
            tunnel: w664 -> [w674 _]
            tunnel: w663 -> [w673 _]
            tunnel: w662 -> [w666 _]
            frame False {
              (unwired) "总分计算"
              n281 = Add(x=w674, y=w673) -> (x+y=w665:i32)
              n282 = Greater Or Equal?(x=w665, y=0) -> (x >= y?=w667:bool)
              n283 = Multiply(x=100, y=w666) -> (x*y=w670:i32)
              n284 = Add(x=w670, y=w665) -> (x+y=w672:i32)
              n285 = To Long Integer(number=w672) -> (32bit integer=w669:i32)
              n286 = case shown="真" w667 {
                tunnel: w669 -> [_ w679]
                frame False {
                  n287 = property on="玩家" class="Str"() -> ("Value"=w675:string)  [unwired: 2 in, 2 out]
                  n288 = Concatenate Strings("亲爱的", w675, "同学，你破产了！游戏结束！") -> (w676:string)
                  n289 = One Button Dialog(message=w676) -> ()  [unwired: 1 in, 1 out]
                }
                frame True {
                  n290 = flat-sequence {
                    tunnel: w679 -> [w682]
                    tunnel: [w683] -> w681
                    tunnel: [w682] -> w680
                    tunnel: w681 -> [w689]
                    tunnel: w680 -> [w688]
                    frame #0 {
                      (unwired) "显示玩家名称与总分"
                      n291 = property on="玩家" class="Str"() -> ("Value"=w683:string)  [unwired: 2 in, 2 out]
                      n292 = Number To Decimal String(number=w682) -> (decimal integer string=w685:string)  [unwired: 1 in]
                      n293 = Concatenate Strings("亲爱的", w683, "同学，经过长期的努力，你挣到了人生的第一桶金！考虑到你的余额、存款、开心值，你的总分为：", w685) -> (w684:string)
                      n294 = One Button Dialog(message=w684) -> ()  [unwired: 1 in, 1 out]
                    }
                    frame #1 {
                      (unwired) "排行榜"
                      n295 = call "rank.vi"("玩家名称"=w689, "得分"=w688) -> ()  [unwired: 1 in]
                    }
                  }
                }
              }
            }
            frame True {
              n296 = property on="玩家" class="Str"() -> ("Value"=w690:string)  [unwired: 2 in, 2 out]
              n297 = Concatenate Strings("亲爱的", w690, "同学，你的健康值低于0，游戏结束！") -> (w691:string)
              n298 = One Button Dialog(message=w691) -> ()  [unwired: 1 in, 1 out]
            }
          }
        }
      }
    }
  }
  n299 = property on="富豪榜" class="MCListbox (严格)"("NumCols"=3, "NumRows"=11) -> ()  [unwired: 2 in, 2 out]
